vi "SwissSPAD Live_Get Firmware Frequency.vi"(8 "Error In":errorcluster, 11 "Firmware Path":path) -> (0 "Error Out":errorcluster, 3 "Frequency (MHz)":i32)   [LabVIEW 2021]
doc: "Looks for a sequence of \"_xx MHz\" in the firmware file path to infer the corresponding trigger frequency in MHz"
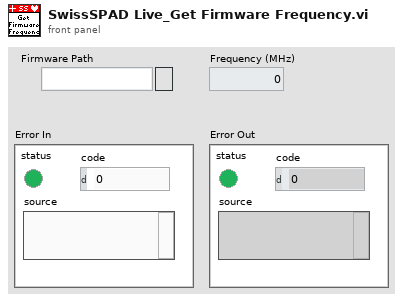
[diagram p1: front panel]
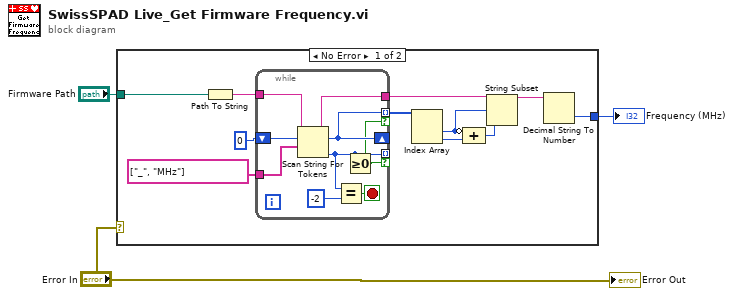
[diagram p0: block diagram]
diagram:
  n1 = case shown="No Error" "Error In" {
    tunnel: [w14 _] -> w3
    tunnel: "Firmware Path" -> [w4 _]
    frame No Error {
      n2 = Path To String(path=w4) -> (string=w5:string)
      n3 = while {
        tunnel: w5 -> [w23]
        tunnel: string[] ["_", "MHz"] ("operators (none)") -> [w22]
        shift-right: [w16] -> _
        shift-left: 0 ("offset past token") -> [w21]
        tunnel: [w18] -> _ mode=indexing if=w15
        tunnel: [w17] -> w9
        tunnel: [w16] -> w8 mode=indexing if=w15
        stop <- w20 stop-if-true
        n4 = Scan String For Tokens(7:w22, 8:w21, 9:w23) -> (0:w18:i32, 2:w16:i32, 3:w17:string)  [unwired: 3 in, 1 out]
        n5 = Equal?(x=w18, y=-2) -> (x = y?=w20:bool)
        n6 = Greater Or Equal To 0?(x=w18) -> (x >= 0?=w15:bool)
      }
      n7 = Index Array(array=w8) -> (element #1=w10:i32, element #2=w11:i32)  [unwired: 2 in]
      n8 = Compound Arithmetic op=ADD(invert w10, w11) -> (w12:i32)
      n9 = String Subset(string=w9, offset (0)=w10, length (rest)=w12) -> (substring=w13:string)
      n10 = Decimal String To Number(string=w13) -> (number=w14:i32)  [unwired: 2 in, 1 out]
    }
    frame Error {
    }
  }
  "Frequency (MHz)" <- w3
  "Error Out" <- "Error In"
